vi "Display.vi"(8 "error in (no error)":errorcluster) -> (0 "error out":errorcluster)   [LabVIEW 2013]
doc: "This VI is an abstraction between the hardware and the simulation"
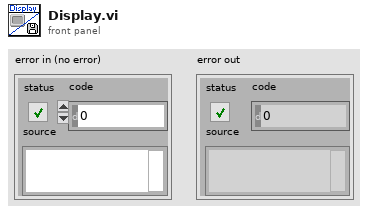
[diagram p1: front panel]
types:
  T1 = typedef "DB_Data.ctl" = cluster{"Door Open Time":dbl, "Travel Time":dbl, "Inactivity Time":dbl, "Door Close Time ":dbl, "Hardware Bit Sensor":T2, "Hardware Bit User console":T2, "Hardware Bit Display":T2, "Controller Bit Display":T2}
  T2 = typedef "Hardware_Enum.ctl" = enum16{"Simulation", "Hardware"}
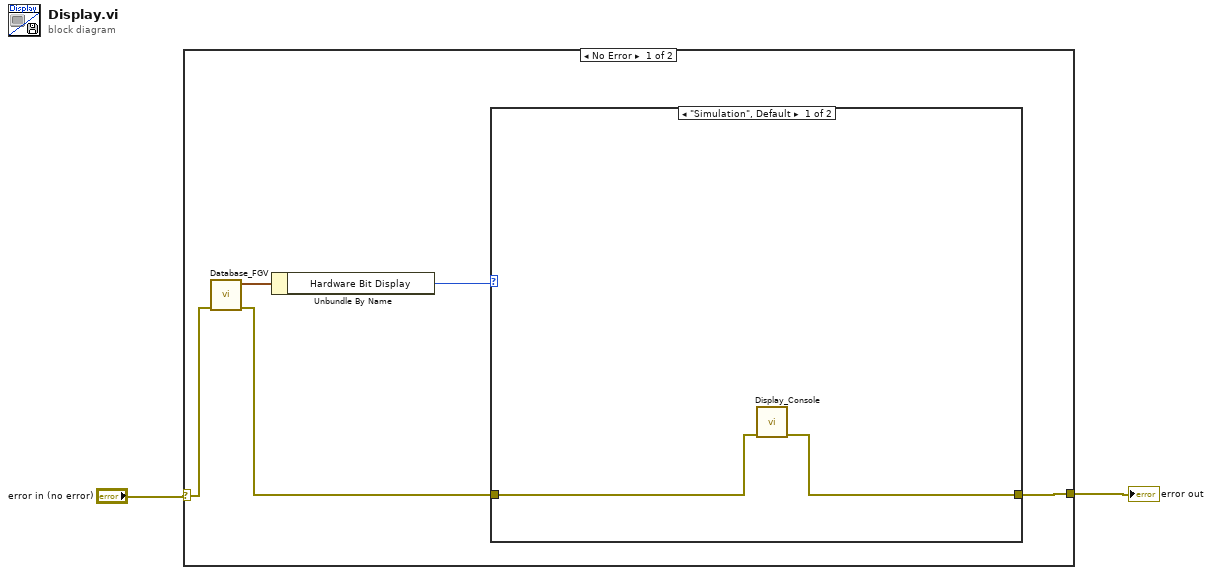
[diagram p0: block diagram]
diagram:
  n1 = case shown="No Error" "error in (no error)" {
    selector: "error in (no error)" -> [w5 w11]
    tunnel: [w4 w11] -> w1
    frame No Error {
      n2 = call "Database_FGV.vi"("error in (no error)"=w5) -> ("error out"=w3:errorcluster, "DB Data Out"=w7:T1)  [unwired: 9 in]
      n3 = Unbundle By Name(w7) -> ("Hardware Bit Display"=w6:T2)
      n4 = case shown="\"Simulation\", Default" w6 {
        tunnel: [w8 w10] -> w4
        tunnel: w3 -> [w9 w10]
        frame "Simulation", Default {
          n5 = call "Display_Console.vi"("error in (no error)"=w9) -> ("error out"=w8:errorcluster)  [unwired: 10 in]
        }
        frame "Hardware" {
          # "Insert Hardware VI here"
        }
      }
    }
    frame Error {
    }
  }
  "error out" <- w1
